vi "PROJECT_ApplicationVersion--constant.vi"() -> (2 "HSE_VERSION_HISTORY":string, 3 "HSE_VERSION_NUMBER":string)   [LabVIEW 2020, in "Project.lvlib"]
doc: "Version number of the application. This is set automatically during build.\n\n____\nHAMPEL SOFTWARE ENGINEERING v2.6.0 (2023-12-19 10:54)"
uses:
  Project.lvlib
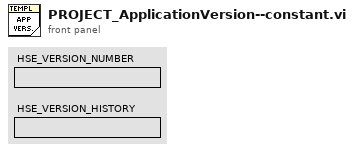
[diagram p1: front panel]
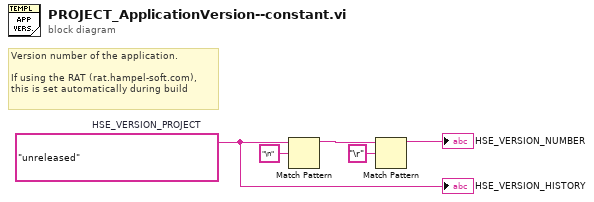
[diagram p0: block diagram]
diagram:
  w4 = "unreleased"  # HSE_VERSION_PROJECT
  # "Version number of the application.\n\nIf using the RAT (rat.hampel-soft.com),\nthis is set automatically during build"
  n1 = Match Pattern(string=w4, regular expression="\n") -> (before substring=w2:string)  [unwired: 1 in, 3 out]
  n2 = Match Pattern(string=w2, regular expression="\r") -> (before substring=→"HSE_VERSION_NUMBER":string)  [unwired: 1 in, 3 out]
  "HSE_VERSION_HISTORY" <- w4
